vi "SendTextMessage.vi"(8 "Body":string, 9 "Subject":string="Vacuum Status!", 10 "phone number":string, 11 "Carrier":enum16{"T-Mobile", "AT&T", "Verizon", "Sprint"}(ring)) -> ()   [LabVIEW 2013]
panel:
  in  "show errors":bool
  in  "smtp server":string="smtp.gmail.com"
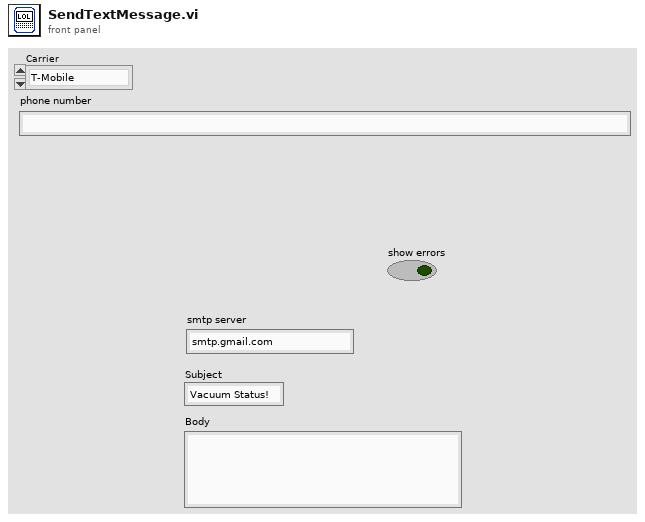
[diagram p1: front panel]
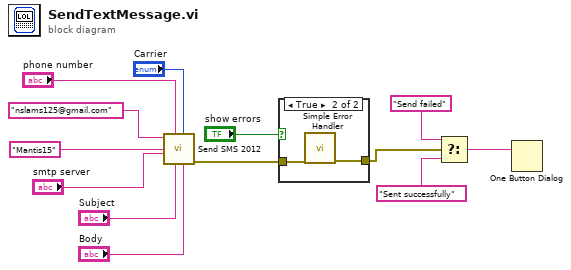
[diagram p0: block diagram]
diagram:
  n1 = call "Send SMS 2012.vi"("Body"="Body", "Carrier"="Carrier", "Subject"="Subject", "phone number"="phone number", "smtp server"="smtp server", "password"="Mantis15", "email username"="nslams125@gmail.com") -> ("Error Out"=w8:errorcluster)  [unwired: 4 in]
  n2 = case shown="True" "show errors" {
    tunnel: w8 -> [w14 w16]
    tunnel: [w14 w15] -> w7
    frame False {
    }
    frame True {
      n3 = call <vilib>:"Simple Error Handler.vi"("error in (no error)"=w16) -> ("error out"=w15:errorcluster)  [unwired: 4 in, 4 out]
    }
  }
  n4 = Select(t="Send failed", s=w7, f="Sent successfully") -> (s? t:f=w9:string)
  n5 = One Button Dialog(message=w9) -> ()  [unwired: 1 in, 1 out]
